vi "Write Characters To File With Err.vi"(4 "convert eol? (no:F)":bool, 6 "append to file? (new file:F)":bool, 8 "error in (no error)":errorcluster, 9 "character string":string, 11 "file path (dialog if empty)":path) -> (0 "error out":errorcluster, 3 "new file path (Not A Path if cancelled)":path)   [LabVIEW 2015]
doc: "LabVIEW no longer supports this VI. Use the Write To Text File function instead. Writes a <B>character string</B> to a new byte stream file or appends the string to an existing file. The VI opens or creates the file before writing to it and closes it afterwards."
uses:
  <vilib>/Utility/error.llb/DialogType.ctl
panel:
  in  "prompt":string="Choose file to write."
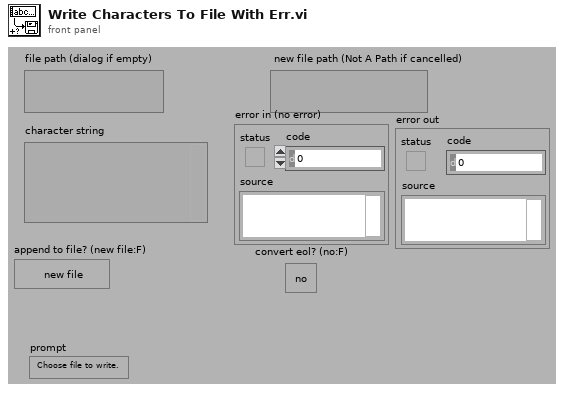
[diagram p1: front panel]
types:
  T1 = typedef "DialogType.ctl" = u16
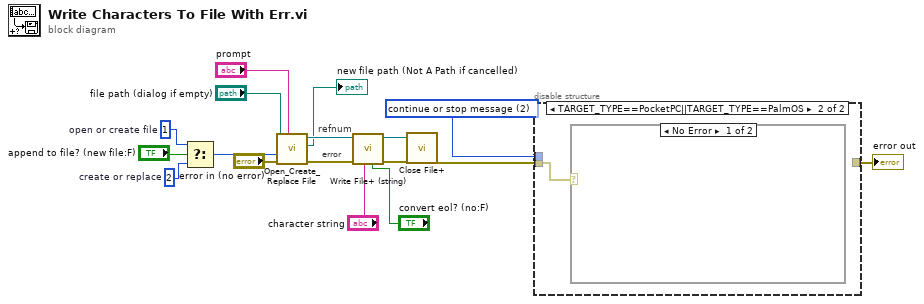
[diagram p0: block diagram]
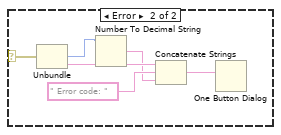
[diagram p3: hidden frame]
diagram:
  w3 = T1 2 items=["no dialog", "OK message", "continue or stop message", "OK message + warnings", "continue/stop + warnings"] ("type of dialog (OK msg:1)")
  w8 = i16 2  # create or replace
  w11 = i16 1  # open or create file
  # "error"
  # "refnum"
  n1 = Select(t=w11, s="append to file? (new file:F)", f=w8) -> (s? t:f=w13:i16)
  n2 = call <vilib>:"Open_Create_Replace File.vi"("prompt"="prompt", "error in (no error)"="error in (no error)", "function (open:0)"=w13, "file path"="file path (dialog if empty)") -> ("error out"=w16:errorcluster, "new file path"=→"new file path (Not A Path if cancelled)":path, "refnum"=w7:refnum<file>)  [unwired: 2 in, 3 out]
  n3 = call <vilib>:"Write File+ (string).vi"("convert eol? (no:F)"="convert eol? (no:F)", "string"="character string", "error in (no error)"=w16, "refnum"=w7) -> ("error out"=w15:errorcluster, "dup refnum"=w14:refnum<file>)  [unwired: 2 in, 2 out]
  n4 = call <vilib>:"Close File+.vi"("error in (no error)"=w15, "refnum"=w14) -> ("error out"=w12:errorcluster)  [unwired: 5 out]
  n5 = disable-structure shown="TARGET_TYPE==PocketPC||TARGET_TYPE==PalmOS" {
    disable-tunnel: w12 -> [w18 w19]
    disable-tunnel: w3 -> [_ _]
    disable-tunnel: [w18 _] -> w2
    frame condition #0 (active) {
    }
    frame condition #1 {
      n6 = case shown="No Error" w19 {
        selector: w19 -> [_ w25]
        frame No Error {
        }
        frame Error {
          n7 = Unbundle(w25) -> ("code"=w24:i32, "source"=w23:string)  [unwired: 1 out]
          n8 = Number To Decimal String(number=w24) -> (decimal integer string=w21:string)  [unwired: 1 in]
          n9 = Concatenate Strings(w23, " Error code: ", w21) -> (w20:string)
          n10 = One Button Dialog(message=w20) -> ()  [unwired: 1 in, 1 out]
        }
      }
    }
  }
  "error out" <- w2
